vi "TestSignalIndex.vi"(6 "initial delay":i32=7, 8 "cycles per sample":i32, 11 "index":i32) -> (0 "valid out":bool, 3 "array index":i32)   [LabVIEW 2013]
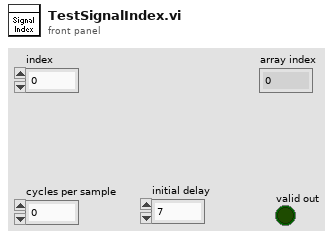
[diagram p1: front panel]
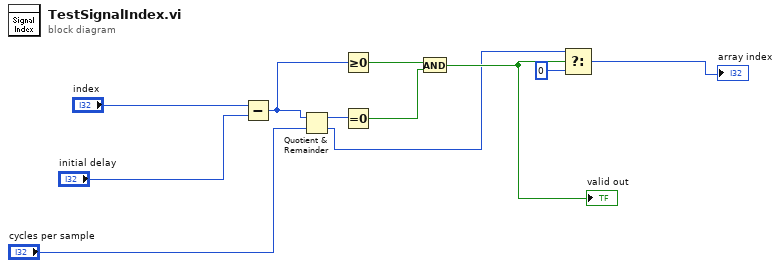
[diagram p0: block diagram]
diagram:
  n1 = Subtract(x="index", y="initial delay") -> (x-y=w7:i32)
  n2 = Quotient & Remainder(x=w7, y="cycles per sample") -> (x-y*floor(x/y)=w11:i32, floor(x/y)=w3:i32)
  n3 = Greater Or Equal To 0?(x=w7) -> (x >= 0?=w6:bool)
  n4 = Equal To 0?(x=w11) -> (x = 0?=w5:bool)
  n5 = And(x=w6, y=w5) -> (x .and. y?=w4:bool)
  "valid out" <- w4
  n6 = Select(t=w3, s=w4, f=0) -> (s? t:f=→"array index":i32)
